vi "Global_Hopper_Disable.vi"() -> ()   [LabVIEW 2017]
panel:
  out "Hopper Disable":bool
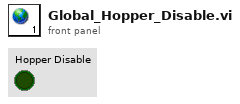
[diagram p1: front panel]
diagram:
